vi "visa.vi"(8 "error in (no error)":errorcluster, 10 "read buffer":string, 11 "Refnum in":T1) -> (0 "error out":errorcluster, 3 "Refnum out":T1)   [LabVIEW 2018]
uses:
  <vilib>/addons/database/Connection.llb/Conn ObjectReference.ctl
  <vilib>/addons/database/NI_Database_API.lvlib
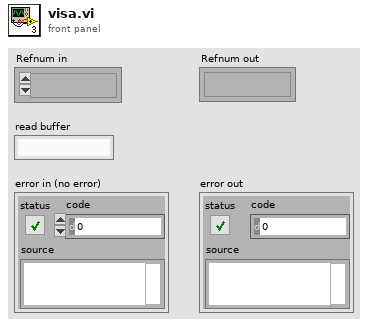
[diagram p1: front panel]
types:
  T1 = typedef "NI_Database_API.lvlib/Conn ObjectReference.ctl" = refnum<k1>
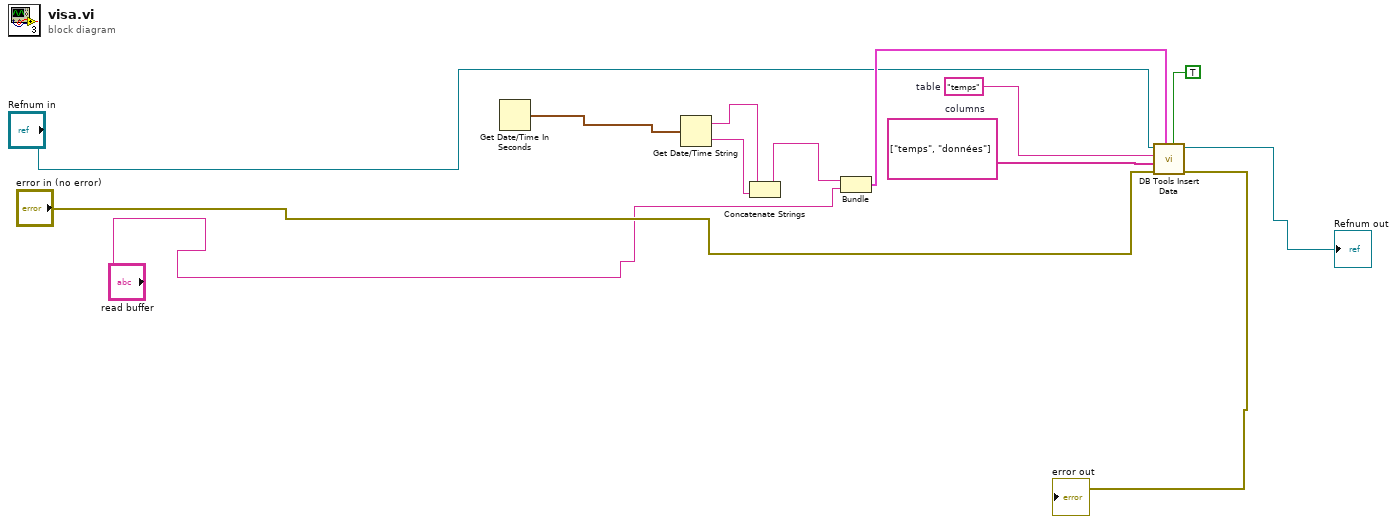
[diagram p0: block diagram]
diagram:
  w9 = string[] ["temps", "données"]  # columns
  w11 = "temps"  # table
  n1 = Get Date/Time In Seconds() -> (seconds since 1Jan1904=w3:timestamp)
  n2 = Get Date/Time String(seconds (now)=w3) -> (date string=w1:string, time string=w2:string)  [unwired: 2 in]
  n3 = Concatenate Strings(w1, w2) -> (w5:string)
  n4 = Bundle(w5, "read buffer"="read buffer") -> (w12:cluster{string, "read buffer":string})  [unwired: 1 in]
  n5 = call <vilib>:"DB Tools Insert Data.vi"("create table? (F)"=TRUE, "data"=w12, "error in (no error)"="error in (no error)", "columns"=w9, "table"=w11, "connection reference"="Refnum in") -> ("error out"=→"error out":errorcluster, "connection reference out"=→"Refnum out":T1)  [unwired: 4 in]
